vi "Calibrate IMU.vi"() -> (2 "Roll bias (deg)":dbl)   [LabVIEW 2021]
uses:
  <vilib>/Platform/TimedLoop/XDataNode/timing_clust.ctl
  <vilib>/Platform/TimedLoop/XDataNode/nitl_modes.ctl
  <vilib>/Platform/TimedLoop/XDataNode/wakeup.ctl
  <vilib>/myRIO/Instrument Drivers/Onboard IO/UART/typedef/VISA Configuration.ctl
  <vilib>/Instr/_visa.llb/VISA Configure Serial Port (Instr).vi
  <vilib>/Platform/TimedLoop/XDataNode/XDataNode.xnode
  <vilib>/myRIO/Express VI/Onboard IO/UART/UART Express VI.xnode
  <vilib>/Platform/TimedLoop/XDataNode/XDNodeRunTimeDep.lvlib
  <vilib>/myRIO/Instrument Drivers/Onboard IO/UART/UART.lvlib
panel:
  in  "UART read period (ms)":dbl=25.0
  out "UART error out":errorcluster
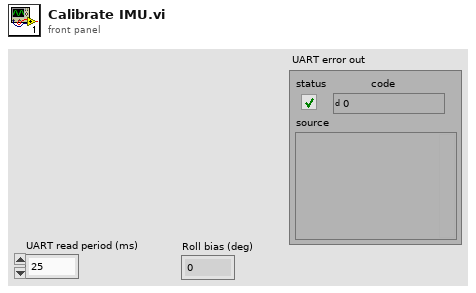
[diagram p1: front panel]
types:
  T1 = typedef "UART.lvlib/VISA Configuration.ctl" = cluster{"baud rate (9600)":u32, "data bits (8)":u16, "parity (0:none)":enum16{"None", "Odd", "Even", "Mark", "Space"}, "stop bits (10: 1 bit)":u16, "flow control (0:none)":u16, "termination char\n(0xA = '\\n' = LF) ":u8, "Enable Termination\nChar (T)":bool, "timeout (10sec)":u32}
  T2 = typedef "XDNodeRunTimeDep.lvlib/timing_clust.ctl" = cluster{"Expected End [f-1]":u64, "Actual End [f-1]":u64, "Finished Late? [f-1]":bool, "Expected End [i-1]":u64, "Actual End [i-1]":u64, "Finished Late? [i-1]":bool, "Expected Start [i]":u64, "Actual Start [i]":u64, "Expected Start [f]":u64, "Actual Start [f]":u64, "Source Name":string, "Structure Name":string, "Period":i64, "Deadline":i64, "Offset":i64, "Start":i64, "Priority":i32, "Timeout":i32, "Mode":T3, "Wakeup Reason":T4, "Error":errorcluster, "Source Type":string, "Secondary Source Type":string, "Global End Time":u64, "Global Start Time":u64, "Frame Duration":u64, "Iteration Duration":u64, "Assigned CPU":i32, "I/O Scan Engine Mode":u32}
  T3 = typedef "XDNodeRunTimeDep.lvlib/nitl_modes.ctl" = enum32{"No Change", "Process missed periods, maintain original phase", "Discard missed periods, maintain original phase", "Process missed periods, ignore original phase", "Discard missed periods, ignore original phase"}
  T4 = typedef "XDNodeRunTimeDep.lvlib/wakeup.ctl" = enum32{"Normal", "Aborted", "Asynchronous wakeup", "Timing source error", "Timed loop error", "Timeout"}
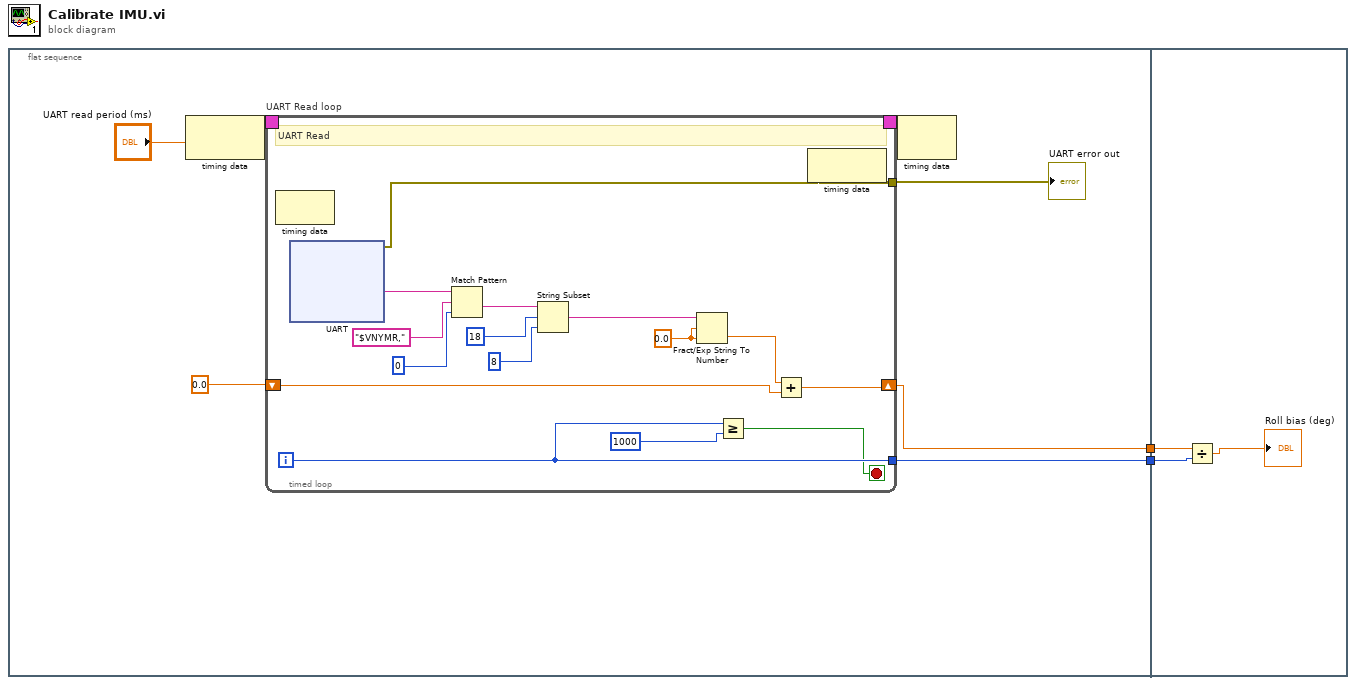
[diagram p0: block diagram]
diagram:
  n1 = flat-sequence {
    tunnel: [w4] -> w2
    tunnel: [w3] -> w1
    tunnel: w2 -> [w50]
    tunnel: w1 -> [w49]
    frame #0 {
      n2 = node-c288("UART read period (ms)") -> (w9:T2)
      n3 = timed-loop "UART Read loop" {
        timing: w9 -> [_]
        timing-out: [_] -> w8
        tunnel: [w18] -> w7
        shift-right: [w15] -> w4
        shift-left: 0.0 -> [w13]
        tunnel: [w11] -> w3
        i -> [w11]
        stop <- w10 stop-if-true
        w16 = 0.0
        # "UART Read"
        n4 = node-c288() -> ()  [unwired: 1 in, 1 out]
        n5 = xnode "UART"() -> ("Characters Read"=w24:string, "error out"=w18:errorcluster)  [unwired: 1 in]
        n6 = Match Pattern(string=w24, regular expression="$VNYMR,", offset (0)=0) -> (after substring=w23:string)  [unwired: 3 out]
        n7 = String Subset(string=w23, offset (0)=18, length (rest)=8) -> (substring=w17:string)
        n8 = Fract/Exp String To Number(string=w17, offset=w16, default (0 dbl)=w16) -> (number=w14:dbl)  [unwired: 1 in, 1 out]
        n9 = Greater Or Equal?(x=w11, y=1000) -> (x >= y?=w10:bool)
        n10 = Add(x=w14, y=w13) -> (x+y=w15:dbl)
        n11 = node-c288() -> ()  [unwired: 1 in, 1 out]
      }
      "UART error out" <- w7
      n12 = node-c288(w8) -> ()  [unwired: 1 out]
    }
    frame #1 {
      n13 = Divide(x=w50, y=w49) -> (x/y=→"Roll bias (deg)":dbl)
    }
  }
